vi "Starter Kit 2.0 Roaming.vi"() -> ()   [LabVIEW 2012]
doc: "This VI demonstrates how to control the Robotics Starter Kit 2.0 robot. It is deployed to an sbRIO-9632, then run on the Real-Time controller."
uses:
  <vilib>/Platform/TimedLoop/XDataNode/timing_clust.ctl
  <vilib>/Platform/TimedLoop/XDataNode/nitl_modes.ctl
  <vilib>/Platform/TimedLoop/XDataNode/wakeup.ctl
  <vilib>/robotics/Starter Kit/2.0/9632 Host Interface/NI_Robotics_Starter Kit Host_9632_2.0.lvclass
  <vilib>/Utility/AngleManip/Degrees to Radians (Scalar DBL).vi
  <vilib>/robotics/Steering/Steering Frame/Apply Steering Frame Velocity to Motors.vi
  <vilib>/Platform/TimedLoop/XDataNode/XDataNode.xnode
  <vilib>/Utility/AngleManip/NI_AngleManipulation.lvlib
  <vilib>/Platform/TimedLoop/XDataNode/XDNodeRunTimeDep.lvlib
  <vilib>/robotics/Steering/Steering Frame/NI_Robotics_Steering Frame.lvclass
  <vilib>/robotics/Starter Kit/Host Interface/NI_Robotics_Starter Kit Host.lvclass
  <vilib>/robotics/Utilities/Scan Angles/NI_Robotics_Scan Angles.lvlib
  <vilib>/robotics/Starter Kit/2.0/NI_Robotics_Starter Kit Host_2.0.lvlib
panel:
  out "Sensor Data":cluster{"angles (deg)":dbl[], "distances":dbl[]}(graph)
  in  "stop":bool
  # "This VI demonstrates how to control the Robotics Starter Kit 2.0 robot. It is deployed to an sbRIO-9632, then run on the Real-Time controller.\n\nInstructions:\n\n1. Set the \"MOTORS\" switch off, then set the \"MASTER\" switch on.  Make sure the robot is connected to the network.\n\n2. Run this VI.  The VI will deploy, and the robot's sensor will start panning left and right.  Accept any prompts to save VIs before deploying.\n\n3. Disconnect the robot from the network so it is no longer tethered.\n\n4. Move the robot to a clear area, then set the \"MOTORS\" switch on.  It will move and avoid obstacles.\n\n5. Set the \"MOTORS\" switch off to shut off power to the motors.\n\n6. Set the \"MASTER\" switch off to shut off power to the entire robot.  You will need to repeat steps 1 through 4 to redeploy after shutting off power*.\n\n*View Starter Kit 2.0 Readme.html for instructions on how to automatically run this VI on startup."
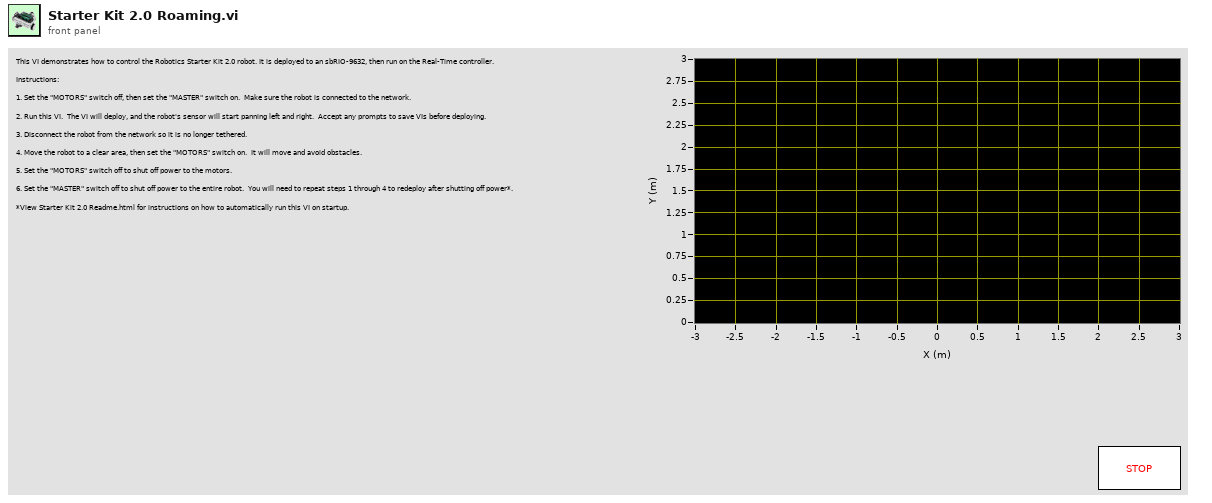
[diagram p1: front panel]
types:
  T1 = typedef "XDNodeRunTimeDep.lvlib/timing_clust.ctl" = cluster{"Expected End [f-1]":u64, "Actual End [f-1]":u64, "Finished Late? [f-1]":bool, "Expected End [i-1]":u64, "Actual End [i-1]":u64, "Finished Late? [i-1]":bool, "Expected Start [i]":u64, "Actual Start [i]":u64, "Expected Start [f]":u64, "Actual Start [f]":u64, "Source Name":string, "Structure Name":string, "Period":i64, "Deadline":i64, "Offset":i64, "Start":i64, "Priority":i32, "Timeout":i32, "Mode":T2, "Wakeup Reason":T3, "Error":errorcluster, "Source Type":string, "Secondary Source Type":string, "Global End Time":u64, "Global Start Time":u64, "Frame Duration":u64, "Iteration Duration":u64, "Assigned CPU":i32, "I/O Scan Engine Mode":u32}
  T2 = typedef "XDNodeRunTimeDep.lvlib/nitl_modes.ctl" = enum32{"No Change", "Process missed periods, maintain original phase", "Discard missed periods, maintain original phase", "Process missed periods, ignore original phase", "Discard missed periods, ignore original phase"}
  T3 = typedef "XDNodeRunTimeDep.lvlib/wakeup.ctl" = enum32{"Normal", "Aborted", "Asynchronous wakeup", "Timing source error", "Timed loop error", "Timeout"}
  T4 = typedef "NI_Robotics_Scan Angles.lvlib/Scan Angle Data.ctl" = cluster{"angles":dbl[], "distances":dbl[], "current index":i32, "previous index":i32}
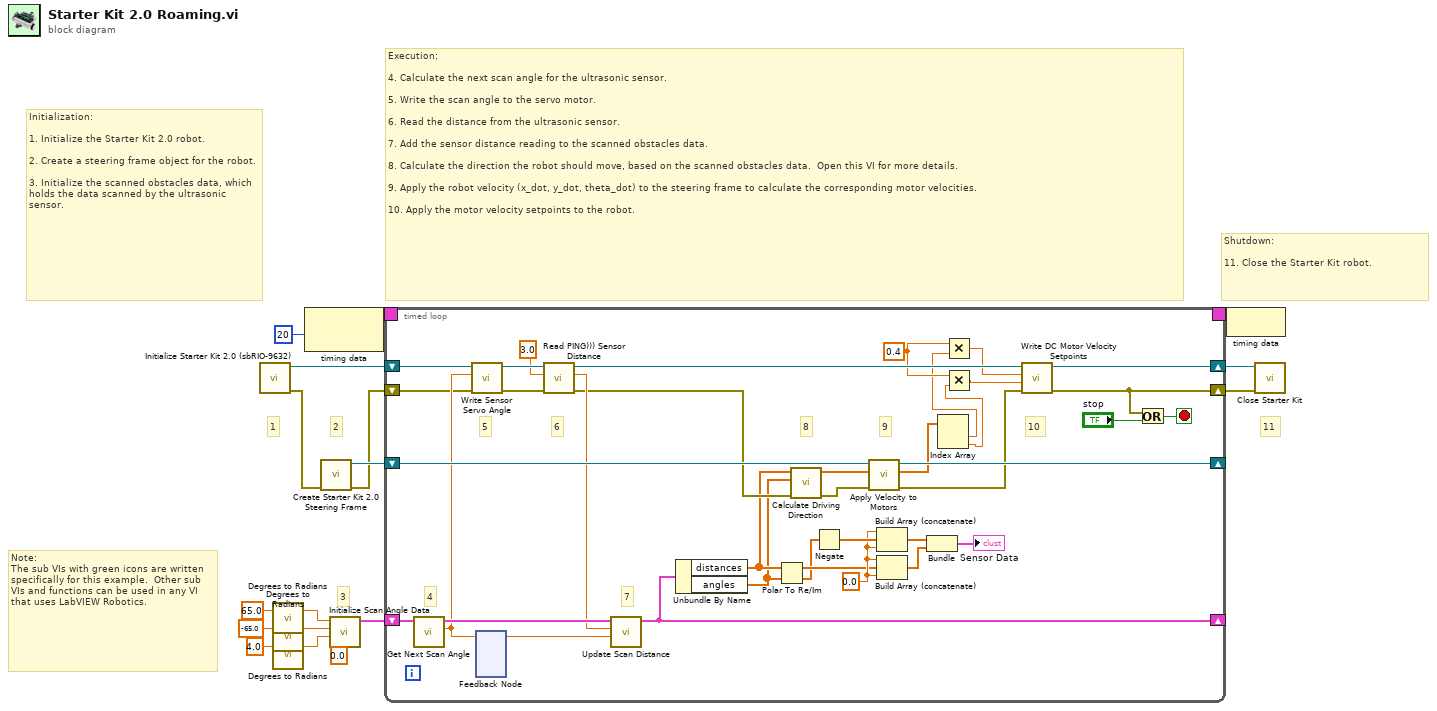
[diagram p0: block diagram]
diagram:
  # "11"
  # "Shutdown:\n\n11. Close the Starter Kit robot."
  # "Execution:\n\n4. Calculate the next scan angle for the ultrasonic sensor.\n\n5. Write the scan angle to the servo motor.\n\n6. Read the distance from the ultrasonic sensor.\n\n7. Add the sensor distance reading to the scanned obstacles data.\n\n8. Calculate the direction the robot should move, based on the scanned obstacles data.  Open this VI for more details.\n\n9. Apply the robot velocity (x_dot, y_dot, theta_dot) to the steering frame to calculate the corresponding motor velocities.\n\n10. Apply the motor velocity setpoints to the robot."
  # "3"
  # "2"
  # "1"
  # "Initialization:\n\n1. Initialize the Starter Kit 2.0 robot.\n\n2. Create a steering frame object for the robot.\n\n3. Initialize the scanned obstacles data, which holds the data scanned by the ultrasonic sensor."
  # "Note:\nThe sub VIs with green icons are written specifically for this example.  Other sub VIs and functions can be used in any VI that uses LabVIEW Robotics."
  n1 = call <vilib>:"Initialize Starter Kit 2.0 (sbRIO-9632).vi"() -> ("error out"=w1:errorcluster, "FPGA starter kit host 2.0 out"=w2:refnum<class "NI_Robotics_Starter Kit Host_9632_2.0.lvclass">)  [unwired: 10 in]
  n2 = call-poly <vilib>:"Degrees to Radians.vi"("angle (deg)"=65.0 ("max angle")) -> ("angle (rad)"=w12:dbl)  [unwired: 2 in]
  n3 = call-poly <vilib>:"Degrees to Radians.vi"("angle (deg)"=-65.0 ("min angle")) -> ("angle (rad)"=w8:dbl)  [unwired: 2 in]
  n4 = call-poly <vilib>:"Degrees to Radians.vi"("angle (deg)"=4.0 ("scan angle")) -> ("angle (rad)"=w9:dbl)  [unwired: 2 in]
  n5 = node-c288(i64 20 ("Period")) -> (w17:T1)
  n6 = call <vilib>:"Create Starter Kit 2.0 Steering Frame.vi"("error in (no error)"=w1) -> ("error out"=w5:errorcluster, "starter kit differential steering frame"=w6:refnum<class "NI_Robotics_Differential Steering Frame.lvclass">)  [unwired: 9 in]
  n7 = call <vilib>:"Initialize Scan Angle Data.vi"("initial angle (0)"=0.0, "scan angle"=w9, "min angle"=w8, "max angle"=w12) -> ("scan angles"=w14:T4)  [unwired: 6 in, 1 out]
  n8 = timed-loop {
    shift-right: [w50] -> _
    shift-left: w14 -> [w52]
    timing: w17 -> [_]
    timing-out: [_] -> w16
    shift-right: [w23] -> w3
    shift-left: w5 -> [w41]
    shift-right: [w38] -> w4
    shift-left: w2 -> [w40]
    shift-right: [w46] -> _
    shift-left: w6 -> [w48]
    stop <- w54 stop-if-true
    w22 = 0.4
    w33 = 0.0 ("element")
    # "10"
    # "9"
    # "8"
    # "7"
    # "6"
    # "5"
    # "4"
    n9 = call <vilib>:"Get Next Scan Angle.vi"("scan angles in"=w52) -> ("new angle"=w44:dbl, "scan angles out"=w51:T4)  [unwired: 9 in]
    n10 = call <vilib>:"Write Sensor Servo Angle.vi"("error in (no error)"=w41, "ccw servo angle (rad)"=w44, "starter kit host in"=w40) -> ("error out"=w25:errorcluster, "starter kit host out"=w26:refnum<class "NI_Robotics_Starter Kit Host_9632_2.0.lvclass">)  [unwired: 7 in]
    n11 = feedback-in #1(w44) -> ()
    n12 = feedback #1() -> (w49:dbl)  [unwired: 1 in]
    n13 = call <vilib>:"Read PING))) Sensor Distance.vi"("error in (no error)"=w25, "default distance (NaN)"=3.0, "starter kit host in"=w26) -> ("error out"=w42:errorcluster, "distance (m)"=w43:dbl, "starter kit host out"=w39:refnum<class "NI_Robotics_Starter Kit Host_9632_2.0.lvclass">)  [unwired: 5 in, 1 out]
    n14 = call <vilib>:"Update Scan Distance.vi"("scan angle"=w49, "new scan distance"=w43, "scan angles in"=w51) -> ("scan angles out"=w50:T4)  [unwired: 8 in]
    n15 = Unbundle By Name(w50) -> ("distances"=w37:dbl[], "angles"=w36:dbl[])
    n16 = Polar To Re/Im(2:w36, 3:w37) -> (0:w30:dbl[], 1:w31:dbl[])
    n17 = call "Calculate Driving Direction.vi"("error in (no error)"=w42, "obstacle angles (rad)"=w36, "obstacle distances (m)"=w37) -> ("error out"=w45:errorcluster, "steering frame velocity"=w47:dbl[])  [unwired: 7 in]
    n18 = Negate(x=w30) -> (-x=w35:dbl[])
    n19 = call-poly <vilib>:"Apply Velocity to Motors.vi"("error in (no error)"=w45, "steering frame velocity"=w47, "steering frame in"=w48) -> ("error out"=w27:errorcluster, "ccw motor velocity setpoints"=w28:dbl[], "steering frame out"=w46:refnum<class "NI_Robotics_Differential Steering Frame.lvclass">)  [unwired: 4 in, 2 out]
    n20 = Build Array (concatenate)(w33, w35, w33) -> (w34:dbl[])
    n21 = Build Array (concatenate)(w33, w31, w33) -> (w32:dbl[])
    n22 = Bundle(w34, w32) -> (→"Sensor Data":cluster{dbl[], dbl[]})  [unwired: 1 in]
    n23 = Index Array(array=w28) -> (element #1=w20:dbl, element #2=w21:dbl)  [unwired: 2 in]
    n24 = Multiply(x=w22, y=w20) -> (x*y=w18:dbl)
    n25 = Multiply(x=w22, y=w21) -> (x*y=w19:dbl)
    n26 = call <vilib>:"Write DC Motor Velocity Setpoints.vi"("error in (no error)"=w27, "right motor ccw velocity (rad/s)"=w19, "left motor ccw velocity (rad/s)"=w18, "starter kit host in"=w39) -> ("error out"=w23:errorcluster, "starter kit host out"=w38:refnum<class "NI_Robotics_Starter Kit Host_9632_2.0.lvclass">)  [unwired: 6 in]
    n27 = Or(x=w23, y="stop") -> (x .or. y?=w54:bool)
  }
  n28 = node-c288(w16) -> ()
  n29 = call-dynamic "Close Starter Kit.vi"("error in (no error)"=w3, "starter kit host in"=w4) -> ()  [unwired: 9 in, 1 out]
